vi "CtoF_SubVI.vi"(1 "Temperatura a Convertir":dbl) -> (0 "Temperatura Convertida":dbl)   [LabVIEW 2013]
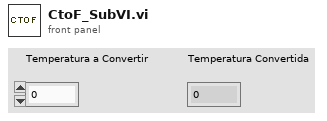
[diagram p1: front panel]
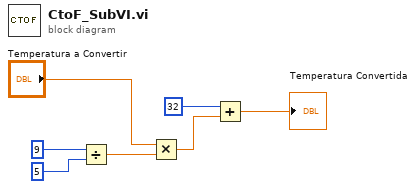
[diagram p0: block diagram]
diagram:
  n1 = Divide(x=9, y=5) -> (x/y=w5:dbl)
  n2 = Multiply(x="Temperatura a Convertir", y=w5) -> (x*y=w4:dbl)
  n3 = Add(x=32, y=w4) -> (x+y=→"Temperatura Convertida":dbl)
